vi "Counter_Angle_V1.vi"() -> ()   [LabVIEW 2015]
panel:
  in  "stop":bool
  out "Crank Angle":dbl
  out "Waveform Chart":dbl(graph)
  out "Gauge":dbl(knob) scale=0.0..360.0
  in  "Encoder PPT":dbl
  in  "Encoder Turn Pulse":bool
  out "RPS Value":dbl
  out "time elapsed in Frame 1":u32
  out "millisecond timer value":u32
  in  "stop 2":bool
  out "Boolean 2":bool
  out "Counts":dbl
  in  "Encoder Rising Simulate":bool
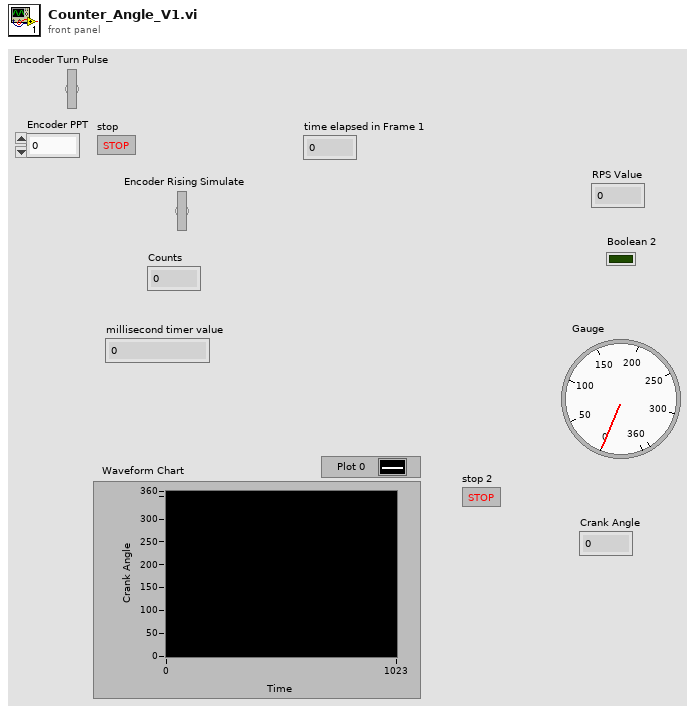
[diagram p1: front panel]
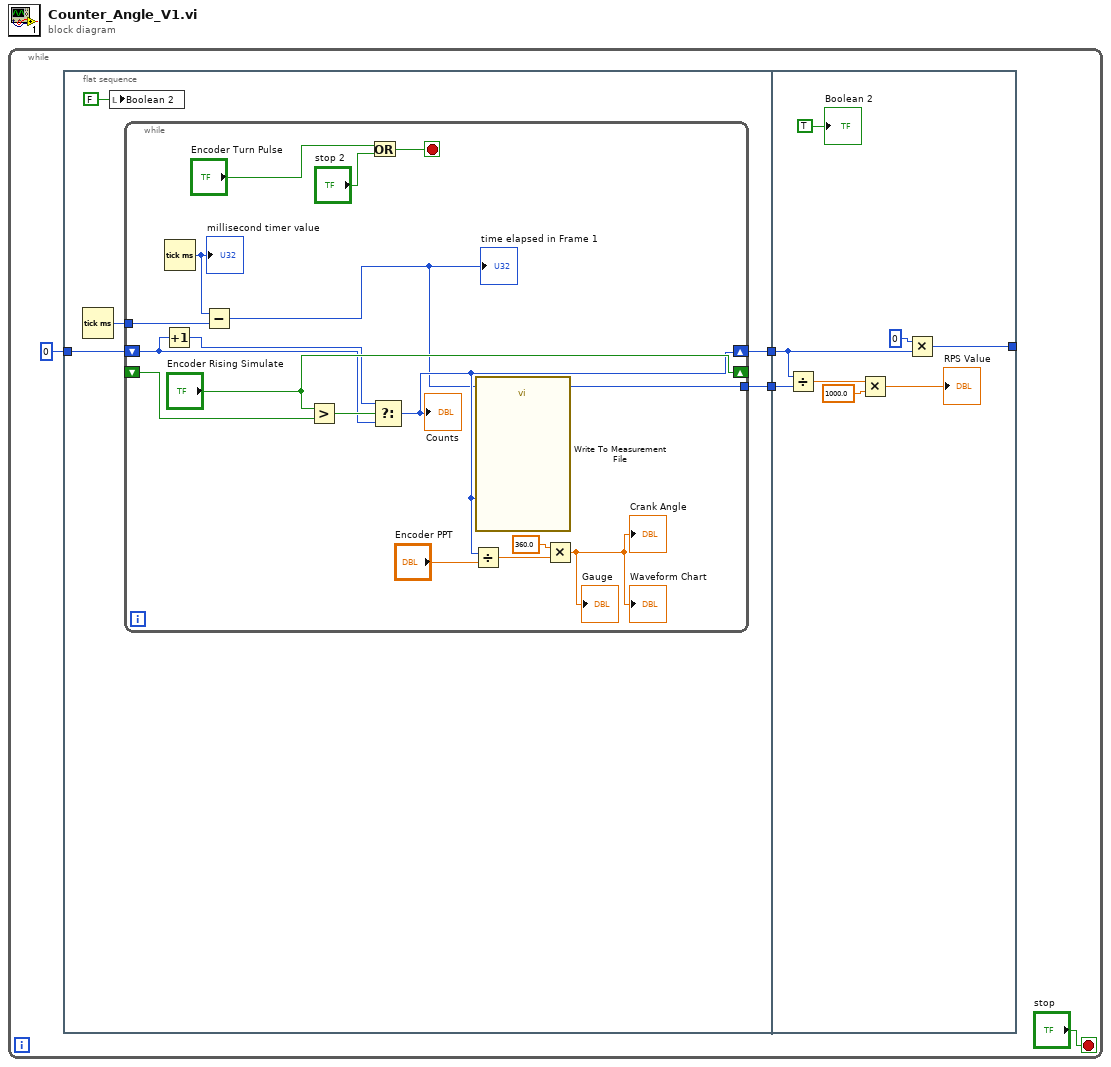
[diagram p0: block diagram]
diagram:
  n1 = while {
    stop <- "stop" stop-if-true
    n2 = flat-sequence {
      tunnel: [w9] -> w4
      tunnel: u8 0 -> [w7]
      tunnel: [w5] -> w2
      tunnel: w4 -> [w26]
      tunnel: w2 -> [w29]
      tunnel: [w28] -> _
      frame #0 {
        n3 = Tick Count (ms)() -> (millisecond timer value=w6:u32)
        n4 = local write "Boolean 2"(FALSE ("Boolean 2")) -> ()
        n5 = while {
          shift-right: ["Encoder Rising Simulate"] -> _
          shift-left: _ -> [w25]
          shift-right: [w11] -> w9
          shift-left: w7 -> [w21]
          tunnel: w6 -> [w19]
          tunnel: [w10] -> w5
          stop <- w13 stop-if-true
          n6 = Increment(x=w21) -> (x+1=w22:u8)
          n7 = Tick Count (ms)() -> (millisecond timer value=w20:u32)
          "millisecond timer value" <- w20
          n8 = Subtract(x=w20, y=w19) -> (x-y=w10:u32)
          "time elapsed in Frame 1" <- w10
          n9 = Greater?(x="Encoder Rising Simulate", y=w25) -> (0:w23:bool)
          n10 = Or(x="Encoder Turn Pulse", y="stop 2") -> (x .or. y?=w13:bool)
          n11 = Select(t=w22, s=w23, f=w21) -> (s? t:f=w11:u8)
          "Counts" <- w11
          n12 = Divide(x=w11, y="Encoder PPT") -> (x/y=w17:dbl)
          n13 = call "Write To Measurement File"("Signals"=w11) -> ()  [unwired: 16 in, 3 out]
          n14 = Multiply(x=360.0, y=w17) -> (x*y=→"Gauge" →"Waveform Chart" →"Crank Angle":dbl)
        }
      }
      frame #1 {
        n15 = Divide(x=w26, y=w29) -> (x/y=w31:dbl)
        n16 = Multiply(x=w31, y=1000.0) -> (x*y=→"RPS Value":dbl)
        n17 = Multiply(x=u8 0, y=w26) -> (x*y=w28:u8)
        "Boolean 2" <- TRUE ("Boolean 2")
      }
    }
  }
